vi "最大似然估计.vi"(1 "sigma":dbl[][](array[numeric]) format="%#_13g", 2 "mu":dbl[][](array[numeric]) format="%#_13g", 3 "pai":dbl[](array[numeric]) format="%#_13g", 4 "cof":dbl[][](array[numeric])) -> (0 "似然距离 2":dbl)   [LabVIEW 2018]
panel:
  out "logMLval":dbl[](array[numeric])
  out "MLval行数":i32
  out "错误输出 3":errorcluster caption="错误输出"
  out "似然估计":dbl[](array[numeric])
  out "sigma大小":i32[](array[numeric])
  out "sigma行数":dbl
  out "输入sigma大小":dbl[](array[numeric])
  out "输入sigma":dbl[][](array[numeric]) format="%#_13g"
  out "错误输出":errorcluster
  out "k":i32
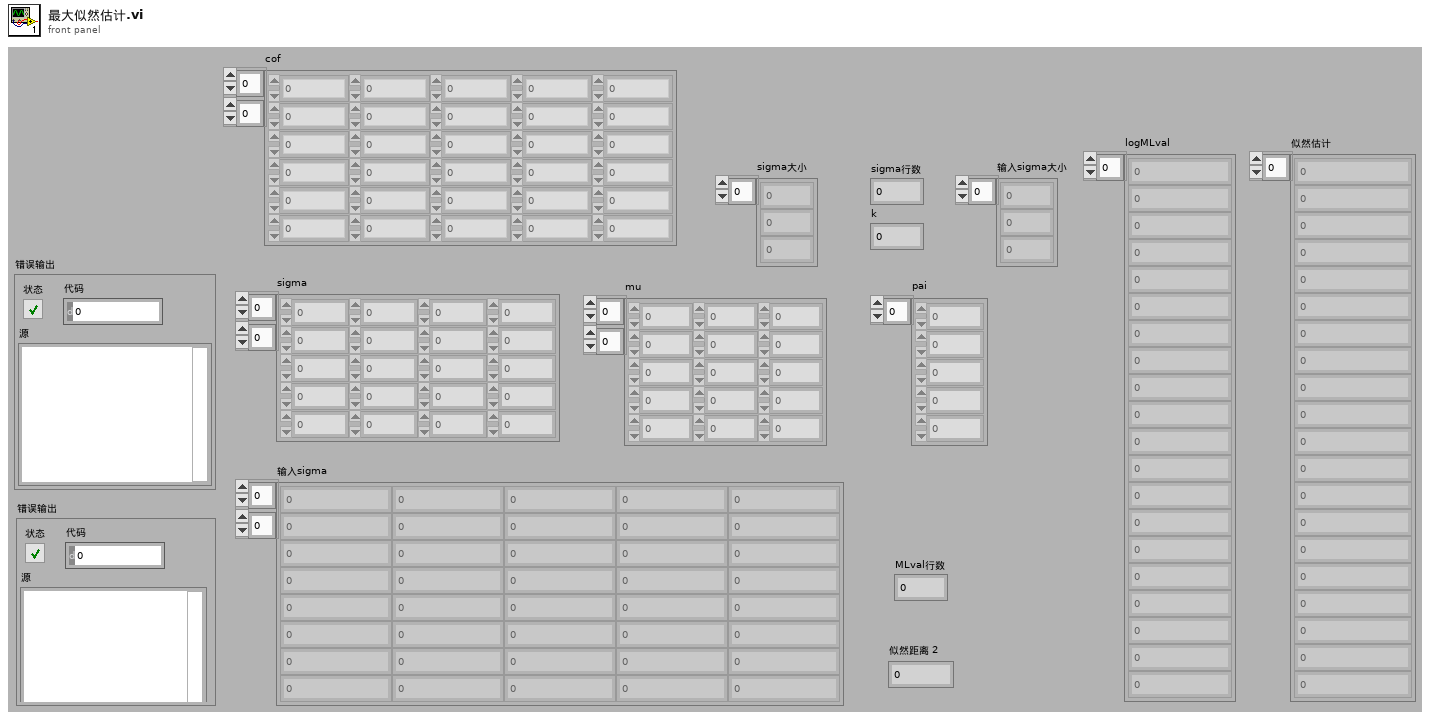
[diagram p1: front panel]
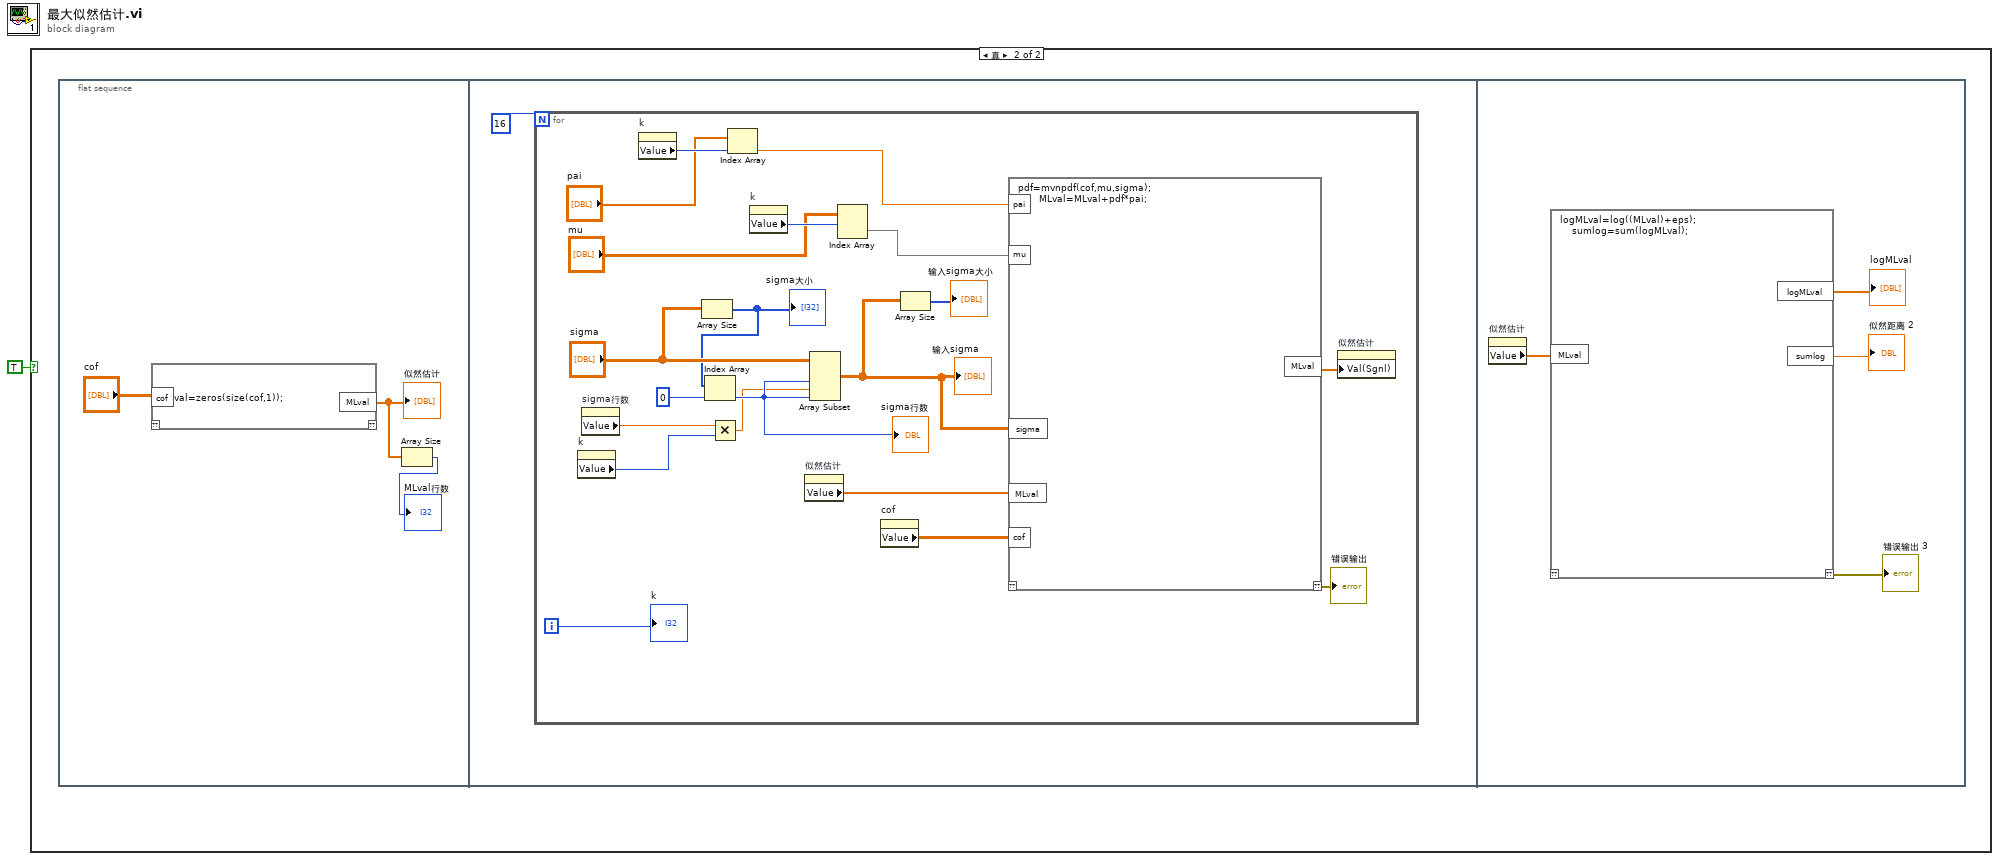
[diagram p0: block diagram]
diagram:
  n1 = case shown="真" TRUE {
    frame False {
    }
    frame True {
      n2 = flat-sequence {
        frame #0 {
          n3 = script code="MLval=zeros(size(cof,1));"("cof"="cof") -> ("MLval"=w3:dbl[])  [unwired: 1 in, 1 out]
          "似然估计" <- w3
          n4 = Array Size(array=w3) -> (size(s)=→"MLval行数":i32)
        }
        frame #1 {
          n5 = for {
            N: 16 -> [_]
            i -> [w15]
            n6 = property on="k" class="DigNum (严格)"() -> ("Value"=w17:i32)  [unwired: 2 in, 2 out]
            n7 = property on="sigma行数" class="DigNum (严格)"() -> ("Value"=w23:dbl)  [unwired: 2 in, 2 out]
            n8 = property on="k" class="DigNum (严格)"() -> ("Value"=w14:i32)  [unwired: 2 in, 2 out]
            n9 = Array Size(array="sigma") -> (size(s)=w19:i32[])
            "sigma大小" <- w19
            n10 = Index Array(array=w19, index=0 ("索引")) -> (element=w24:i32)
            "sigma行数" <- w24
            n11 = Multiply(x=w23, y=w17) -> (x*y=w18:dbl)
            n12 = Index Array(array="pai", index=w14) -> (element=w12:dbl)
            n13 = property on="k" class="DigNum (严格)"() -> ("Value"=w11:i32)  [unwired: 2 in, 2 out]
            n14 = property on="似然估计" class="Arr (严格)"() -> ("Value"=w6:dbl[])  [unwired: 2 in, 2 out]
            n15 = Array Subset(array="sigma", length (row)=w24, index (col)=w18, length (col)=w24) -> (w16:dbl[][])  [unwired: 1 in]
            "输入sigma" <- w16
            n16 = Index Array(array="mu", index (row)=w11) -> (element=w9:dbl[])  [unwired: 1 in]
            n17 = property on="cof" class="Arr (严格)"() -> ("Value"=w8:dbl[][])  [unwired: 2 in, 2 out]
            n18 = Array Size(array=w16) -> (size(s)=→"输入sigma大小":i32[])
            n19 = script code="pdf=mvnpdf(cof,mu,sigma);\n       MLval=MLval+pdf*pai;"("pai"=w12, "mu"=w9, "sigma"=w16, "cof"=w8, "MLval"=w6) -> ("??"=→"错误输出":errorcluster, "MLval"=w7:dbl[])  [unwired: 1 in]
            n20 = property on="似然估计" class="Arr (严格)"("Val(Sgnl)"=w7) -> ()  [unwired: 2 in, 2 out]
            "k" <- w15
          }
        }
        frame #2 {
          n21 = property on="似然估计" class="Arr (严格)"() -> ("Value"=w27:dbl[])  [unwired: 2 in, 2 out]
          n22 = script code="logMLval=log((MLval)+eps);\n    sumlog=sum(logMLval);"("MLval"=w27) -> ("??"=→"错误输出 3":errorcluster, "sumlog"=→"似然距离 2":dbl, "logMLval"=→"logMLval":dbl[])  [unwired: 1 in]
        }
      }
    }
  }
